vi "WriteCmd.vi"(1 "error IO":errorcluster, 2 "Command":string, 3 "VISA resource name":refnum<visa-resource-name>) -> (0 "error":errorcluster)   [LabVIEW 2010]
doc: "This VI flushes the transmit buffer and transmits a command.\nNote that the input command need not contain CR LF because those characters are concatenated onto the input string.\nNote that 40, the integer argument for VISA Flush I/O Buffer,s is hexadecimal."
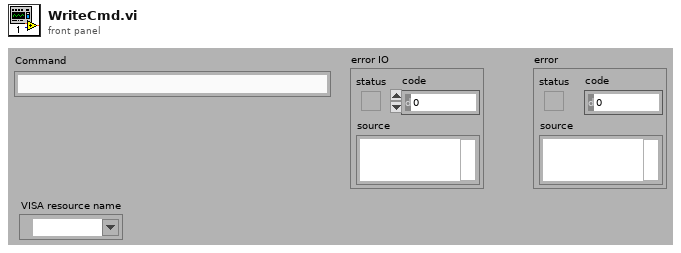
[diagram p1: front panel]
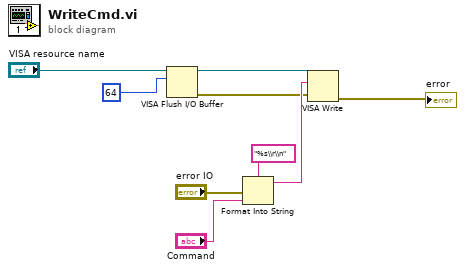
[diagram p0: block diagram]
diagram:
  n1 = VISA Flush I/O Buffer(VISA resource name="VISA resource name", mask (16)=u16 64) -> (VISA resource name out=w3:refnum<visa-resource-name>, error out=w2:errorcluster)  [unwired: 1 in]
  n2 = Format Into String "Format Into String"(format string="%s\\r\\n", error in="error IO", "Command") -> (resulting string=w7:string)  [unwired: 1 in, 1 out]
  n3 = VISA Write(VISA resource name=w3, write buffer=w7, error in (no error)=w2) -> (error out=→"error":errorcluster)  [unwired: 2 out]
